vi "Get Function Code.vi"(8 "error in":errorcluster, 11 "CANopen Msg in":refnum<class "CANopen Message.lvclass">) -> (0 "error out":errorcluster, 2 "Function Code":T1 items=["NMT"=0, "EMCY/SYNC"=1, "TIME"=2, "PDO1 (tx)"=3, "PDO1 (rx)"=4, "PDO2 (tx)"=5, "PDO2 (rx)"=6, "PDO3 (tx)"=7, "PDO3 (rx)"=8, "PDO4 (tx)"=9, "PDO4 (rx)"=10, "SDO (tx)"=11, "SDO (rx)"=12, "NMT error control"=14], 3 "CANopen Msg out":refnum<class "CANopen Message.lvclass">)   [LabVIEW 2020, in "CANopen.lvlib" / "CANopen Message.lvclass"]
uses:
  CANopen Message.lvclass
  CANopen Message.lvclass/CANopen Message.ctl
  Typedefs/Function Code.ctl
  CANopen.lvlib
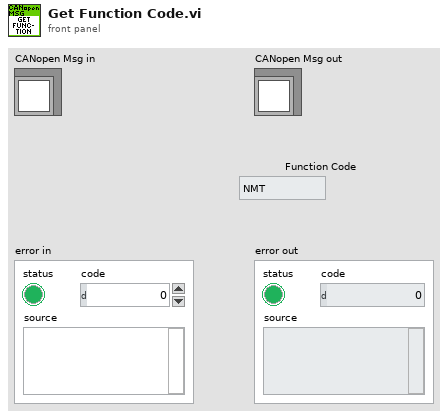
[diagram p1: front panel]
types:
  T1 = typedef "CANopen.lvlib/Function Code.ctl" = u8
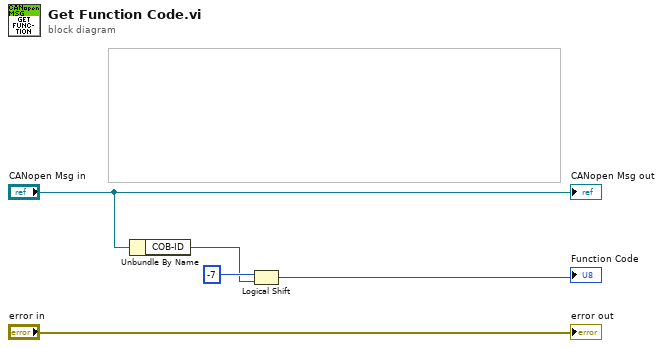
[diagram p0: block diagram]
diagram:
  n1 = Unbundle By Name("CANopen Msg in") -> ("COB-ID"=w2:u32)
  n2 = Logical Shift(y=i16 -7, x=w2) -> (x << y=→"Function Code":u32)
  "CANopen Msg out" <- "CANopen Msg in"
  "error out" <- "error in"
